vi "Calculate adjusted frame period.vi"() -> (1 "Frame rate set OR original (fps)":dbl, 3 "Original frame period (ms)":i32, 5 "Original frame rate (fps)":dbl)   [LabVIEW 2013]
uses:
  Globals/gl_Time series viewer globals.vi
panel:
  out "New frame rate (fps)":dbl
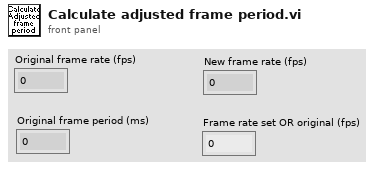
[diagram p1: front panel]
types:
  T1 = typedef "AVI playback header info cluster.ctl" = cluster{"Frame Size":u32, "AOD fill time (us)":dbl, "Dwell time (us)":dbl, "Frame period (ms)":dbl, "Number of Miniscans":u16, "Number of Pixels in Miniscan":u16}
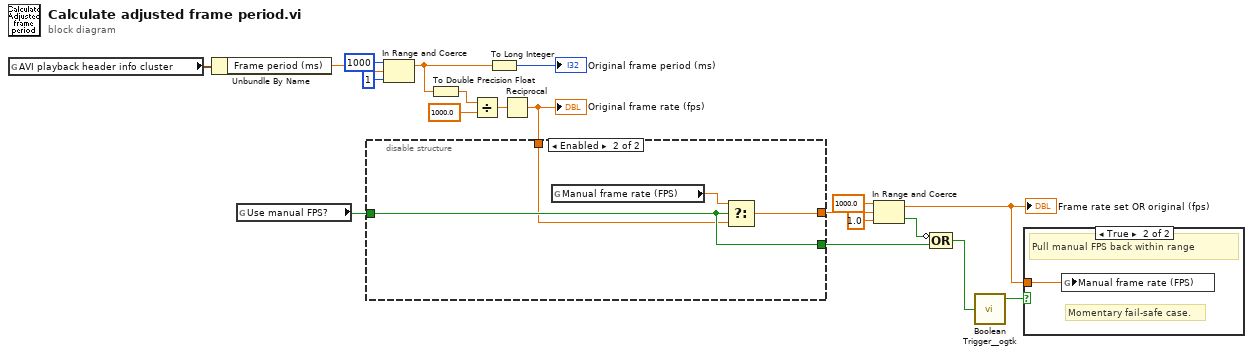
[diagram p0: block diagram]
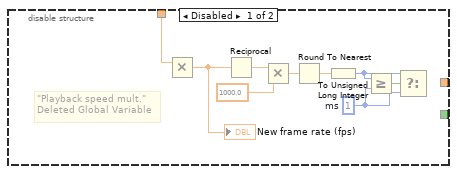
[diagram p3: hidden frame]
diagram:
  n1 = global read "gl_Time series viewer globals.vi" "AVI playback header info cluster"() -> (w16:T1)
  n2 = Unbundle By Name(w16) -> ("Frame period (ms)"=w2:dbl)
  n3 = global read "gl_Time series viewer globals.vi" "Use manual FPS?"() -> (w15:bool)
  n4 = In Range and Coerce(upper limit=u32 1000, x=w2, lower limit=u32 1) -> (coerced(x)=w1:dbl)  [unwired: 1 out]
  n5 = To Double Precision Float(number=w1) -> (double precision float=w17:dbl)
  n6 = Divide(x=w17, y=1000.0) -> (x/y=w7:dbl)
  n7 = To Long Integer(number=w1) -> (32bit integer=→"Original frame period (ms)":i32)
  n8 = Reciprocal(x=w7) -> (1/x=w18:dbl)
  "Original frame rate (fps)" <- w18
  n9 = disable-structure shown="Enabled" {
    disable-tunnel: w18 -> [w28 w29]
    disable-tunnel: w15 -> [_ w31]
    disable-tunnel: [_ w31] -> w11
    disable-tunnel: [_ w30] -> w6
    frame Disabled {
      w21 = u32 1  # ms
      # "\"Playback speed mult.\"\nDeleted Global Variable"
      n10 = Multiply(x=w28) -> (x*y=w20:dbl)  [unwired: 1 in]
      "New frame rate (fps)" <- w20
      n11 = Reciprocal(x=w20) -> (1/x=w27:dbl)
      n12 = Multiply(x=w27, y=1000.0) -> (x*y=w25:dbl)
      n13 = Round To Nearest(number=w25) -> (nearest integer value=w23:dbl)
      n14 = To Unsigned Long Integer(number=w23) -> (unsigned 32bit integer=w22:u32)
      n15 = Greater Or Equal?(x=w22, y=w21) -> (x >= y?=w24:bool)
      n16 = Select(t=w22, s=w24, f=w21) -> ()  [unwired: 1 out]
    }
    frame Enabled {
      n17 = global read "gl_Time series viewer globals.vi" "Manual frame rate (FPS)"() -> (w32:dbl)
      n18 = Select(t=w32, s=w31, f=w29) -> (s? t:f=w30:dbl)
    }
  }
  n19 = In Range and Coerce(upper limit=1000.0, x=w6, lower limit=1.0) -> (coerced(x)=w8:dbl, In Range?=w12:bool)
  "Frame rate set OR original (fps)" <- w8
  n20 = Compound Arithmetic op=OR(invert w12, w11) -> (w10:bool)
  n21 = call "Boolean Trigger__ogtk.vi"("Boolean Input"=w10) -> ("Rising Edge"=w9:bool)  [unwired: 1 in, 1 out]
  n22 = case shown="True" w9 {
    tunnel: w8 -> [_ w33]
    frame False {
    }
    frame True {
      # "Momentary fail-safe case."
      # "Pull manual FPS back within range"
      n23 = global write "gl_Time series viewer globals.vi" "Manual frame rate (FPS)"(w33) -> ()
    }
  }
